vi "Flip Flop T (2).vi"(10 "Q1":bool, 11 "T":bool) -> (3 "Boolean":bool)   [LabVIEW 2018]
panel:
  in  "stop":bool
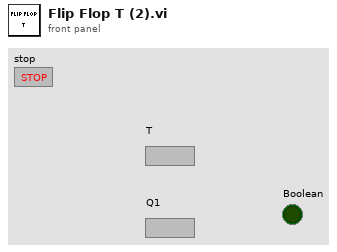
[diagram p1: front panel]
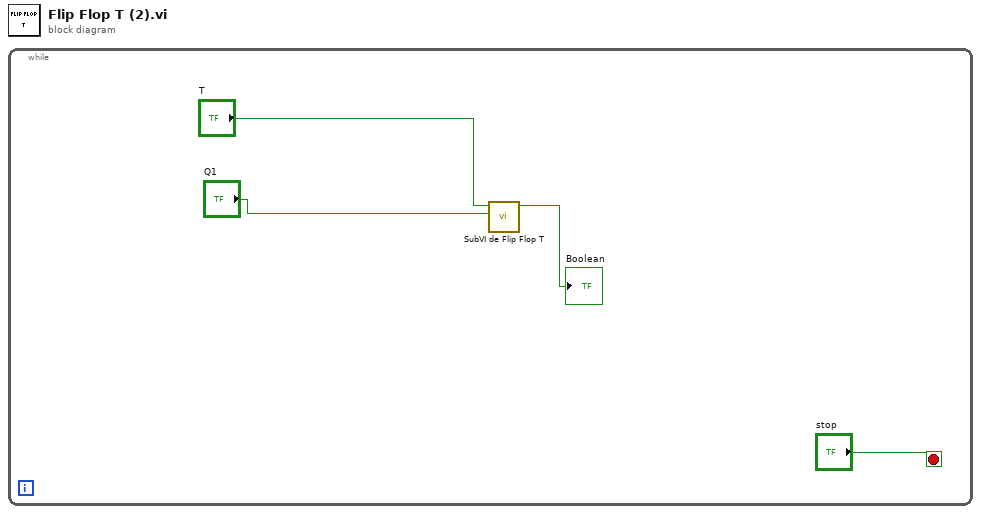
[diagram p0: block diagram]
diagram:
  n1 = while {
    stop <- "stop" stop-if-true
    n2 = call "SubVI de Flip Flop T.vi"("Q1"="Q1", "T"="T") -> ("Q1*"=→"Boolean":bool)  [unwired: 9 in]
  }
